vi "hse-application__GetSingleton.vi"(11 "Action":T1=enum."Get") -> (0 "Error Out":errorcluster, 3 "ApplicationClass DVR":refnum<data-value>)   [LabVIEW 2022 SP3, in "hse-application.lvclass"]
doc: "Contains the DVR to the HSE ApplicationClass object.\n\n____\nHAMPEL SOFTWARE ENGINEERING v3.8.0 (2023-12-18 14:41)"
uses:
  hse-application.lvclass
  hse-misc/Controls/FGV_Actions.ctl
  hse-application.lvclass/hse-application.ctl
  hse-misc/hse-misc.lvlib
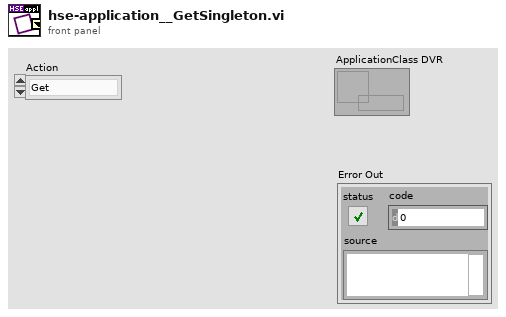
[diagram p1: front panel]
types:
  T1 = typedef "hse-misc.lvlib/FGV_Actions.ctl" = enum16{"Set", "Get"}
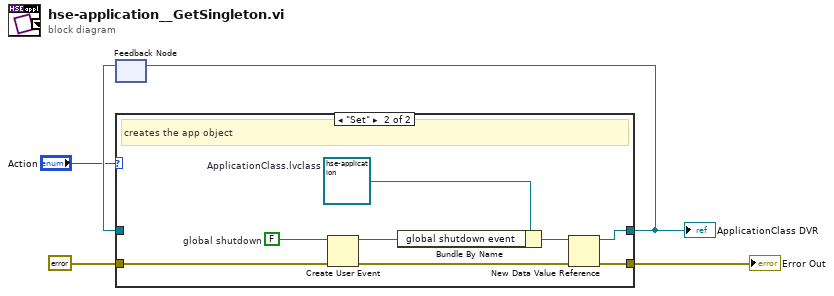
[diagram p0: block diagram]
diagram:
  n1 = feedback #1() -> (w4:refnum<data-value>)  [unwired: 1 in]
  n2 = case shown="\"Set\"" "Action" {
    tunnel: [w7 w15] -> w5
    tunnel: w4 -> [w7 _]
    tunnel: [w6 w14] -> w2
    tunnel: errorcluster {"status"=FALSE, "code"=0, "source"=""} ("error out") -> [w6 w8]
    frame Default {
      # "returns an existing object"
    }
    frame "Set" {
      w13 = FALSE  # global shutdown
      w11 = refnum<class "hse-application.lvclass"> refnum  # ApplicationClass.lvclass
      # "creates the app object"
      n3 = Create User Event(user event datatype=w13, error in=w8) -> (user event=w12:refnum<user-event>, error out=w9:errorcluster)
      n4 = Bundle By Name(cluster=w11, "global shutdown event"=w12) -> (w10:refnum<class "hse-application.lvclass">)
      n5 = New Data Value Reference(data value=w10, error in=w9) -> (data value reference=w15:refnum<data-value>, error out=w14:errorcluster)
    }
  }
  "ApplicationClass DVR" <- w5
  "Error Out" <- w2
  n6 = feedback-in #1(w5) -> ()
